vi "AWG Initialize.vi"(8 "error in (no error)":errorcluster, 9 "Reset (True)":bool=TRUE, 10 "ID Query (True)":bool=TRUE, 11 "awg session in":T1) -> (0 "error out":errorcluster, 2 "idn string":string, 3 "awg session out":T1)   [LabVIEW 2018, in "AWG.lvlib"]
doc: "AWG wrapper: initialize function generator."
uses:
  AWG.lvlib
  AWG Session.ctl
  AWG Type.ctl
  Agilent 33XXX Series/Agilent 33XXX Series.lvlib
  Agilent 3352X Series/Agilent 3352X Series.lvlib
  AFG3000/Tektronix AFG 3000 Series.lvlib
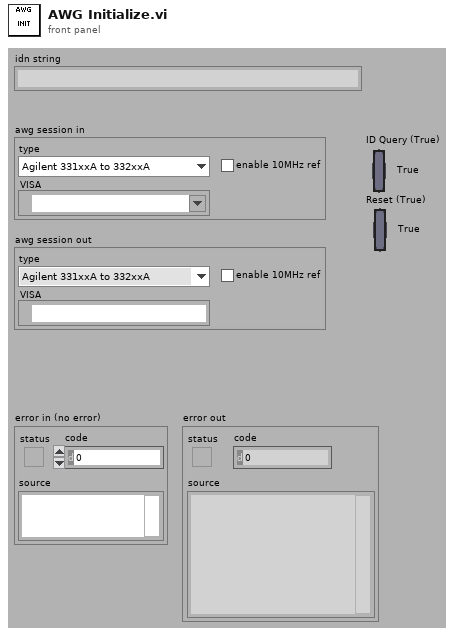
[diagram p1: front panel]
types:
  T1 = typedef "AWG.lvlib/AWG Session.ctl" = cluster{"type":T2, "VISA":refnum<visa-resource-name>, "enable 10MHz ref":bool}
  T2 = typedef "AWG.lvlib/AWG Type.ctl" = enum16{"Agilent 331xxA to 332xxA", "Agilent 335xxA to 336xxA", "Tektronix AFG3101C", "dummy"}
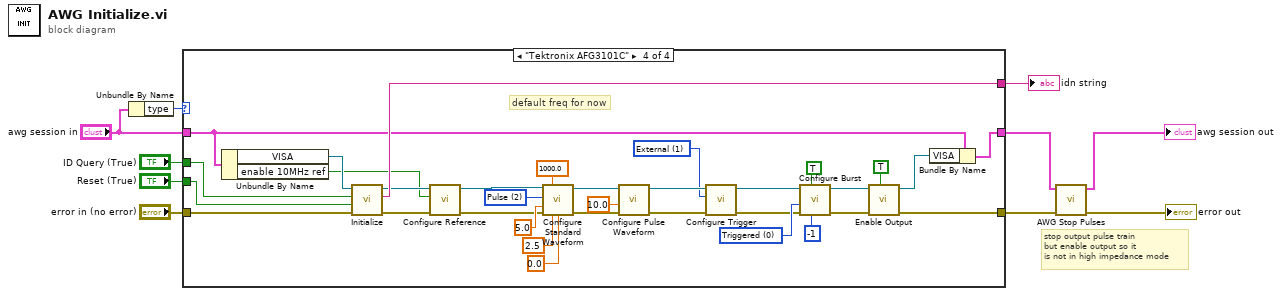
[diagram p0: block diagram]
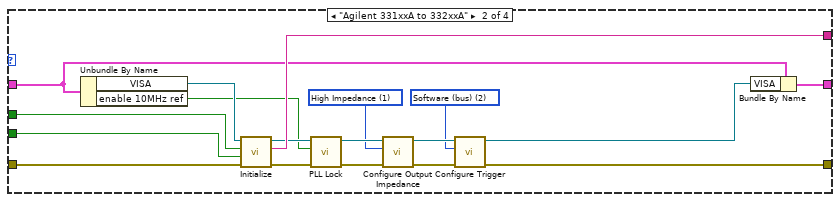
[diagram p3: hidden frame]
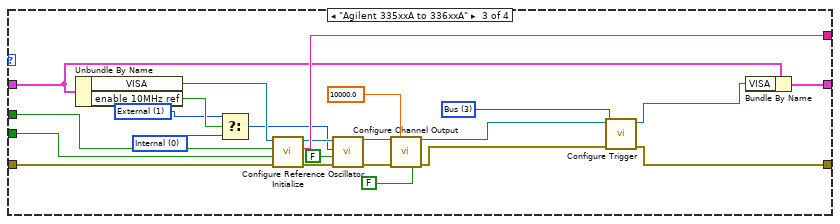
[diagram p4: hidden frame]
diagram:
  # "stop output pulse train\nbut enable output so it \nis not in high impedance mode"
  n1 = Unbundle By Name("awg session in") -> ("type"=w10:T2)
  n2 = case shown="\"Tektronix AFG3101C\"" w10 {
    tunnel: "error in (no error)" -> [w12 w30 w53 w86]
    tunnel: [_ w29 w52 w82] -> w8
    tunnel: [w12 w13 w32 w69] -> w4
    tunnel: "awg session in" -> [w11 w26 w50 w68]
    tunnel: [w11 w27 w49 w66] -> w2
    tunnel: "ID Query (True)" -> [_ w25 w45 w84]
    tunnel: "Reset (True)" -> [_ w24 w44 w85]
    frame Default {
    }
    frame "Agilent 331xxA to 332xxA" {
      w15 = u16 2 items=["Internal", "External", "Software (bus)"] ("Trigger Source (0: Internal)")
      w18 = u16 1 items=["50 Ohms", "High Impedance", "User Defined"] ("Impedance (0: 50 Ohms)")
      n3 = Unbundle By Name(w26) -> ("VISA"=w28:refnum<visa-resource-name>, "enable 10MHz ref"=w21:bool)
      n4 = call "Initialize.vi"("error in (no error)"=w30, "Reset (True)"=w24, "ID Query (True)"=w25, "VISA resource name"=w28) -> ("error out"=w23:errorcluster, "idn string"=w29:string, "VISA resource name out"=w22:refnum<visa-resource-name>)  [unwired: 5 in]
      n5 = call "PLL Lock.vi"("error in (no error)"=w23, "PLL lock  (T: Enable)"=w21, "VISA resource name"=w22) -> ("error out"=w20:errorcluster, "VISA resource name out"=w19:refnum<visa-resource-name>)  [unwired: 7 in]
      n6 = call "Configure Output Impedance.vi"("error in (no error)"=w20, "Impedance (0: 50 Ohms)"=w18, "VISA resource name"=w19) -> ("error out"=w17:errorcluster, "VISA resource name out"=w16:refnum<visa-resource-name>)  [unwired: 7 in]
      n7 = call "Configure Trigger.vi"("error in (no error)"=w17, "Trigger Source (0: Internal)"=w15, "VISA resource name"=w16) -> ("error out"=w13:errorcluster, "VISA resource name out"=w14:refnum<visa-resource-name>)  [unwired: 7 in]
      n8 = Bundle By Name(cluster=w26, "VISA"=w14) -> (w27:T1)
    }
    frame "Agilent 335xxA to 336xxA" {
      w31 = 3 items=["Immediate", "External", "Timer", "Bus"] ("Trigger Source (0: Immediate)")
      w37 = 1 items=["Internal", "External"] ("Source (0: Internal)")
      w36 = 0 items=["Internal", "External"] ("Source (0: Internal)")
      n9 = Unbundle By Name(w50) -> ("VISA"=w51:refnum<visa-resource-name>, "enable 10MHz ref"=w46:bool)
      n10 = Select(t=w37, s=w46, f=w36) -> (s? t:f=w38:i32)
      n11 = call "Initialize.vi"("error in (no error)"=w53, "Reset (Enable)"=w44, "ID Query (Enable)"=w45, "VISA resource name"=w51) -> ("error out"=w47:errorcluster, "idn string"=w52:string, "VISA resource name out"=w48:refnum<visa-resource-name>)  [unwired: 5 in]
      n12 = call "Configure Reference Oscillator.vi"("error in (no error)"=w47, "Source Auto Selection(T: Enable)"=FALSE, "Source (0: Internal)"=w38, "VISA resource name"=w48) -> ("error out"=w43:errorcluster, "VISA resource name out"=w42:refnum<visa-resource-name>)  [unwired: 6 in]
      n13 = call "Configure Channel Output.vi"("VISA resource name"=w42, "Output Impedance (50 Ohm)"=10000.0, "error in (no error)"=w43, "Enable Voltage Limit (T: Enable)"=FALSE) -> ("VISA resource name out"=w35:refnum<visa-resource-name>, "error out"=w33:errorcluster)  [unwired: 10 in]
      n14 = call "Configure Trigger.vi"("error in (no error)"=w33, "Trigger Source (0: Immediate)"=w31, "VISA resource name"=w35) -> ("error out"=w32:errorcluster, "VISA resource name out"=w34:refnum<visa-resource-name>)  [unwired: 7 in]
      n15 = Bundle By Name(cluster=w50, "VISA"=w34) -> (w49:T1)
    }
    frame "Tektronix AFG3101C" {
      w54 = u16 1 items=["Internal"=3, "External"=1] ("Trigger Source (3:Internal)")
      w73 = u16 0 items=["Triggered", "Gated"] ("Burst Mode (0: Triggered)")
      w78 = u16 2 items=["Sine", "Square", "Pulse", "Ramp", "Noise", "DC", "Sin(x)/x", "Gaussian", "Lorentz", "Exponential Rise", "Exponential Decay", "Haversine"] ("Waveform Function (0: Sine)")
      # "default freq for now"
      n16 = Unbundle By Name(w68) -> ("VISA"=w83:refnum<visa-resource-name>, "enable 10MHz ref"=w60:bool)
      n17 = call "Initialize.vi"("error in (no error)"=w86, "Reset (True)"=w85, "ID Query (True)"=w84, "VISA resource name"=w83) -> ("error out"=w64:errorcluster, "idn string"=w82:string, "VISA resource name out"=w63:refnum<visa-resource-name>)  [unwired: 5 in]
      n18 = call "Configure Reference.vi"("error in (no error)"=w64, "external clock"=w60, "VISA resource name"=w63) -> ("error out"=w62:errorcluster, "VISA resource name out"=w61:refnum<visa-resource-name>)  [unwired: 7 in]
      n19 = call "Configure Standard Waveform.vi"("VISA resource name"=w61, "Frequency (1000 Hz)"=1000.0, "Waveform Function (0: Sine)"=w78, "Amplitude (1 Vpp)"=5.0, "error in (no error)"=w62, "DC Offset (0.00 V)"=2.5, "Phase Level (-1)"=0.0) -> ("VISA resource name out"=w75:refnum<visa-resource-name>, "error out"=w76:errorcluster)  [unwired: 7 in]
      n20 = call "Configure Pulse Waveform.vi"("error in (no error)"=w76, "Duty Cycle (50%)"=10.0, "VISA resource name"=w75) -> ("error out"=w58:errorcluster, "VISA resource name out"=w55:refnum<visa-resource-name>)  [unwired: 7 in]
      n21 = call "Configure Trigger.vi"("error in (no error)"=w58, "Trigger Source (3:Internal)"=w54, "VISA resource name"=w55) -> ("error out"=w57:errorcluster, "VISA resource name out"=w56:refnum<visa-resource-name>)  [unwired: 7 in]
      n22 = call "Configure Burst.vi"("Burst Count (5)"=-1, "Enable Burst (T: Enable)"=TRUE, "error in (no error)"=w57, "Burst Mode (0: Triggered)"=w73, "VISA resource name"=w56) -> ("error out"=w71:errorcluster, "VISA resource name out"=w70:refnum<visa-resource-name>)  [unwired: 5 in]
      n23 = call "Enable Output.vi"("Enable Output (T: Enable)"=TRUE, "error in (no error)"=w71, "VISA resource name"=w70) -> ("error out"=w69:errorcluster, "VISA resource name out"=w67:refnum<visa-resource-name>)  [unwired: 7 in]
      n24 = Bundle By Name(cluster=w68, "VISA"=w67) -> (w66:T1)
    }
  }
  "idn string" <- w8
  n25 = call "AWG Stop Pulses.vi"("error in (no error)"=w4, "awg session in"=w2) -> ("error out"=→"error out":errorcluster, "awg session out"=→"awg session out":T1)  [unwired: 8 in]
